vi "Refresh UI.vi"(8 "error in (no error)":errorcluster, 11 "Main in":refnum<class "Main.lvclass">) -> (0 "error out":errorcluster, 3 "Main out":refnum<class "Main.lvclass">)   [LabVIEW 2020, in "Main.lvclass"]
uses:
  Main.lvclass
  Main.lvclass/Main.ctl
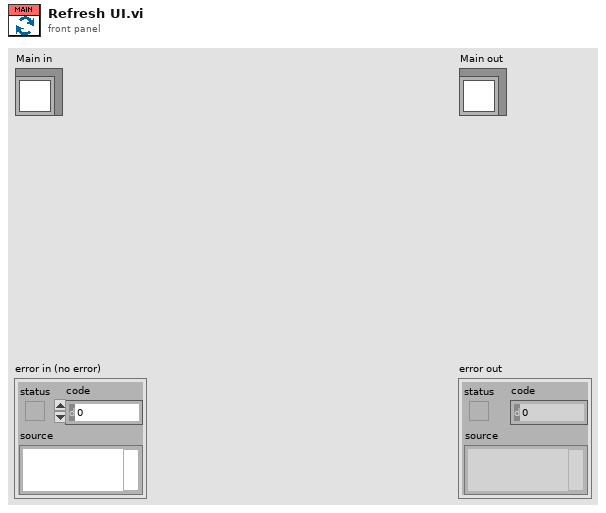
[diagram p1: front panel]
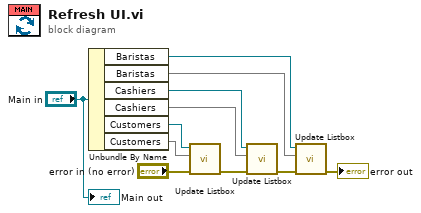
[diagram p0: block diagram]
diagram:
  n1 = Unbundle By Name("Main in") -> ("Baristas"=w8:refnum<vi>, "Baristas"=w10:map{string, string}, "Cashiers"=w7:refnum<vi>, "Cashiers"=w4:map{string, string}, "Customers"=w6:refnum<vi>, "Customers"=w5:map{string, string})
  n2 = call "Update Listbox.vi"("error in (no error)"="error in (no error)", "Status Map"=w5, "MulticolumnListbox Reference In"=w6) -> ("error out"=w3:errorcluster)  [unwired: 7 in, 1 out]
  n3 = call "Update Listbox.vi"("error in (no error)"=w3, "Status Map"=w4, "MulticolumnListbox Reference In"=w7) -> ("error out"=w1:errorcluster)  [unwired: 7 in, 1 out]
  n4 = call "Update Listbox.vi"("error in (no error)"=w1, "Status Map"=w10, "MulticolumnListbox Reference In"=w8) -> ("error out"=→"error out":errorcluster)  [unwired: 7 in, 1 out]
  "Main out" <- "Main in"
